vi "Convert from Seconds.vi"(1 "Time Unit":T1(ring), 2 "Seconds":dbl format="%.2f") -> (0 "Quantity":dbl format="%.2f")   [LabVIEW 2014]
doc: "This VI converts the entered value from seconds to a user specified time unit."
panel:
  # "Select Help»Show Context Help and move the cursor over the VI icon to display help for this VI."
  # "Enter a number of seconds to calculate the equivalent quantity in the specified time unit."
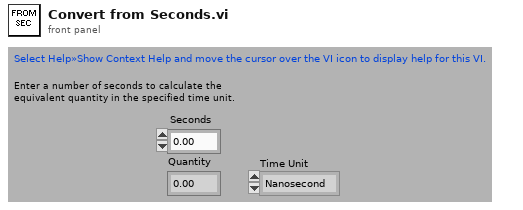
[diagram p1: front panel]
types:
  T1 = enum16{"Nanosecond", "Microsecond", "Millisecond", "Second", "Minute", "Hour", "Day", "Week", "Month", "Year", "Decade", "Century", "Millennium"}
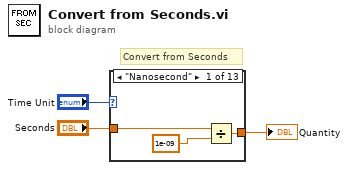
[diagram p0: block diagram]
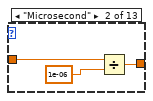
[diagram p2: hidden frame]
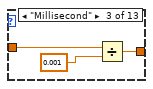
[diagram p3: hidden frame]
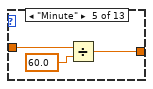
[diagram p5: hidden frame]
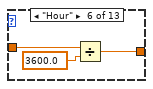
[diagram p6: hidden frame]
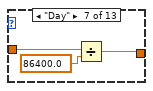
[diagram p7: hidden frame]
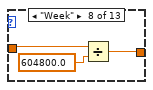
[diagram p8: hidden frame]
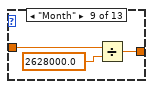
[diagram p9: hidden frame]
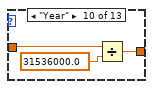
[diagram p10: hidden frame]
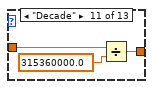
[diagram p11: hidden frame]
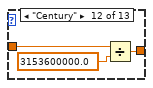
[diagram p12: hidden frame]
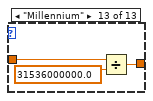
[diagram p13: hidden frame]
diagram:
  # "Convert from Seconds"
  n1 = case shown="\"Nanosecond\"" "Time Unit" {
    tunnel: "Seconds" -> [w4 w7 w10 w13 w16 w18 w22 w25 w27 w29 w33 w35 w38]
    tunnel: [w5 w8 w11 w13 w14 w17 w20 w23 w26 w30 w32 w36 w39] -> w1
    frame "Nanosecond" {
      n2 = Divide(x=w4, y=1e-09) -> (x/y=w5:dbl)
    }
    frame "Microsecond" {
      n3 = Divide(x=w7, y=1e-06) -> (x/y=w8:dbl)
    }
    frame "Millisecond" {
      n4 = Divide(x=w10, y=0.001) -> (x/y=w11:dbl)
    }
    frame "Second", Default {
    }
    frame "Minute" {
      n5 = Divide(x=w16, y=60.0) -> (x/y=w14:dbl)
    }
    frame "Hour" {
      n6 = Divide(x=w18, y=3600.0) -> (x/y=w17:dbl)
    }
    frame "Day" {
      n7 = Divide(x=w22, y=86400.0) -> (x/y=w20:dbl)
    }
    frame "Week" {
      n8 = Divide(x=w25, y=604800.0) -> (x/y=w23:dbl)
    }
    frame "Month" {
      n9 = Divide(x=w27, y=2628000.0) -> (x/y=w26:dbl)
    }
    frame "Year" {
      n10 = Divide(x=w29, y=31536000.0) -> (x/y=w30:dbl)
    }
    frame "Decade" {
      n11 = Divide(x=w33, y=315360000.0) -> (x/y=w32:dbl)
    }
    frame "Century" {
      n12 = Divide(x=w35, y=3153600000.0) -> (x/y=w36:dbl)
    }
    frame "Millennium" {
      n13 = Divide(x=w38, y=31536000000.0) -> (x/y=w39:dbl)
    }
  }
  "Quantity" <- w1
